vi "Motors Manual IO.vi"(2 "error in":errorcluster, 3 "Emergency Stop Reference":refnum<vi>, 4 "VISA in":refnum<visa-resource-name>="COM7") -> (0 "error out":errorcluster, 1 "VISA out":refnum<visa-resource-name>="COM7")   [LabVIEW 2018]
uses:
  <vilib>/Utility/error.llb/DialogType.ctl
panel:
  in  "stop":bool
  in  "Read":bool
  in  "Write Buffer":string="1QM"
  out "Error Code: Read":i32 format="%0.0f"
  out "Error Source: Read":string
  out "Error Message: Read":string=" INSTRUCTIONS:\r\rNormal Use:  When using subVIs that incorporate the error in/error out (or error I/O) structure, place this handler where you want to inform the user of an error, typically at the end of the I/O data path, as the last action of the program.  If the error in error? is ERROR, the handler creates a message describing the error and its source.  If the type of dialog = 1 (default), the message is displayed to the user, who can only acknowedge it.  If the type = 2, the user can acknowledge the message or abort execution; aborting a program with active I/O is not recommended.  If the type = 0, no message is displayed; this is used to process the error programmatically, and the error out cluster elements are wired to individual terminals for that reason.  \r\rOther Use:\n\r\nlocal testing.  To test the error code of a subVI or function that does not have the error I/O structure, you can wire its error code and a source string to the local error code and error source inputs.  If error in error? indicates no error and error code is not equal to 0, the local code and source are substituted for the error in values, and error? is set TRUE (ERROR)."
  out "Error Message: Write":string=" INSTRUCTIONS:\r\rNormal Use:  When using subVIs that incorporate the error in/error out (or error I/O) structure, place this handler where you want to inform the user of an error, typically at the end of the I/O data path, as the last action of the program.  If the error in error? is ERROR, the handler creates a message describing the error and its source.  If the type of dialog = 1 (default), the message is displayed to the user, who can only acknowedge it.  If the type = 2, the user can acknowledge the message or abort execution; aborting a program with active I/O is not recommended.  If the type = 0, no message is displayed; this is used to process the error programmatically, and the error out cluster elements are wired to individual terminals for that reason.  \r\rOther Use:\n\r\nlocal testing.  To test the error code of a subVI or function that does not have the error I/O structure, you can wire its error code and a source string to the local error code and error source inputs.  If error in error? indicates no error and error code is not equal to 0, the local code and source are substituted for the error in values, and error? is set TRUE (ERROR)."
  out "Error Source: Write":string
  out "Error Code: Write":i32 format="%0.0f"
  in  "Write":bool
  out "Read Buffer":string
  # "Note that this subVI monopolizes the motor I/O.  Press \"Close Window\" before attempting to send motor commands in the main VI."
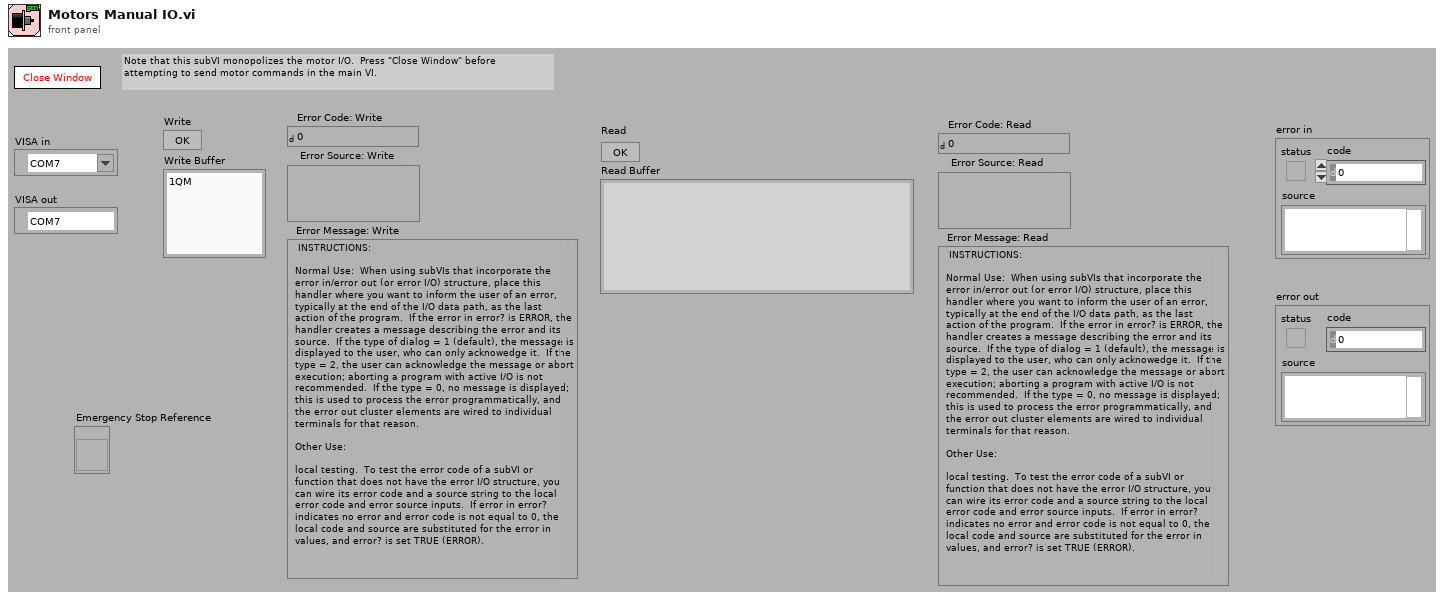
[diagram p1: front panel]
types:
  T1 = typedef "DialogType.ctl" = u16
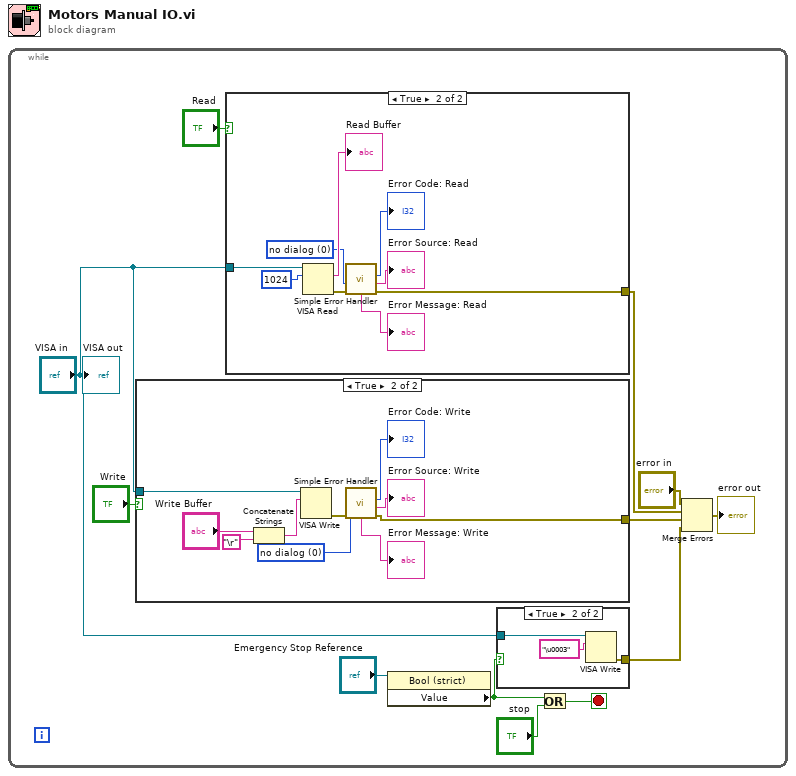
[diagram p0: block diagram]
diagram:
  n1 = while {
    stop <- w6 stop-if-true
    n2 = case shown="True" "Write" {
      tunnel: "VISA in" -> [_ w34]
      tunnel: [_ w26] -> w9
      frame False {
      }
      frame True {
        w25 = T1 0 items=["no dialog", "OK message", "continue or stop message", "OK message + warnings", "continue/stop + warnings"] ("type of dialog (OK msg:1)")
        n3 = Concatenate Strings("Write Buffer", "\r") -> (w31:string)
        n4 = VISA Write(VISA resource name=w34, write buffer=w31) -> (error out=w30:errorcluster)  [unwired: 1 in, 2 out]
        n5 = call <vilib>:"Simple Error Handler.vi"("type of dialog (OK msg:1)"=w25, "error in (no error)"=w30) -> ("code out"=→"Error Code: Write":i32, "source out"=→"Error Source: Write":string, "error out"=w26:errorcluster, "message"=→"Error Message: Write":string)  [unwired: 3 in, 1 out]
      }
    }
    n6 = case shown="True" "Read" {
      tunnel: "VISA in" -> [_ w22]
      tunnel: [_ w17] -> w10
      frame False {
      }
      frame True {
        w16 = T1 0 items=["no dialog", "OK message", "continue or stop message", "OK message + warnings", "continue/stop + warnings"] ("type of dialog (OK msg:1)")
        n7 = VISA Read(VISA resource name=w22, byte count=u32 1024) -> (read buffer=→"Read Buffer":string, error out=w18:errorcluster)  [unwired: 1 in, 2 out]
        n8 = call <vilib>:"Simple Error Handler.vi"("type of dialog (OK msg:1)"=w16, "error in (no error)"=w18) -> ("code out"=→"Error Code: Read":i32, "source out"=→"Error Source: Read":string, "error out"=w17:errorcluster, "message"=→"Error Message: Read":string)  [unwired: 3 in, 1 out]
      }
    }
    n9 = property on="Property Node" class="Bool (strict)"(reference="Emergency Stop Reference") -> ("Value"=w4:bool)  [unwired: 1 in, 2 out]
    n10 = case shown="True" w4 {
      tunnel: "VISA in" -> [_ w15]
      tunnel: [_ w13] -> w1
      frame False {
      }
      frame True {
        n11 = VISA Write(VISA resource name=w15, write buffer="\u0003") -> (error out=w13:errorcluster)  [unwired: 1 in, 2 out]
      }
    }
    n12 = Or(x=w4, y="stop") -> (x .or. y?=w6:bool)
    n13 = Merge Errors("error in", w10, w9, w1) -> (→"error out":errorcluster)
    "VISA out" <- "VISA in"
  }
